vi "Test Assert In SubVI.vi"(8 "error in (no error)":errorcluster) -> (0 "error out":errorcluster)   [LabVIEW 2009]
uses:
  classes/Assert/Assert.lvclass
  classes/Test/Test.lvclass
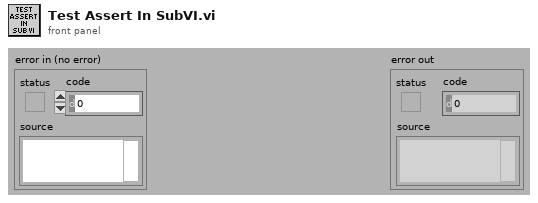
[diagram p1: front panel]
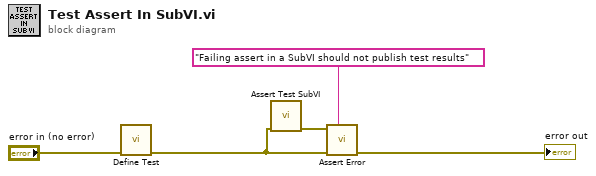
[diagram p0: block diagram]
diagram:
  n1 = call "Define Test.vi"("error in (no error)"="error in (no error)") -> ("error out"=w1:errorcluster)  [unwired: 10 in]
  n2 = call "Assert Test SubVI.vi"("error in (no error)"=w1) -> ("error out"=w3:errorcluster)  [unwired: 10 in]
  n3 = call "Assert Error.vi"("Label"="Failing assert in a SubVI should not publish test results", "error in (no error)"=w1, "Error?"=w3) -> ("error out"=→"error out":errorcluster)  [unwired: 8 in]
